vi "Write_Realim_Current.vi"(9 "Objetive Current":dbl, 11 "address string in":string) -> (1 "Boolean":bool, 3 "address string in 2":string)   [LabVIEW 2017]
panel:
  out "error out":errorcluster
  out "Numeric":i32
  out "Correction(x)":dbl
  out "Current":dbl[unit]
  out "Offset":dbl
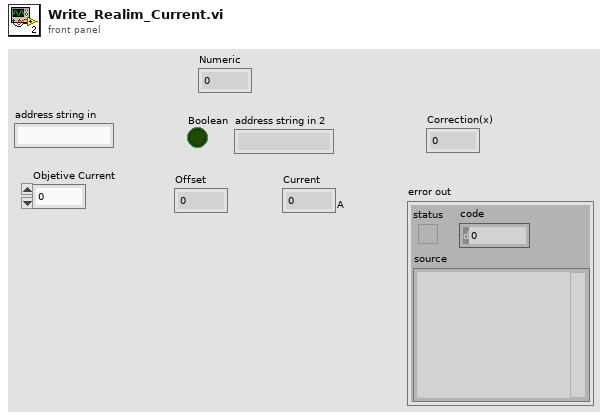
[diagram p1: front panel]
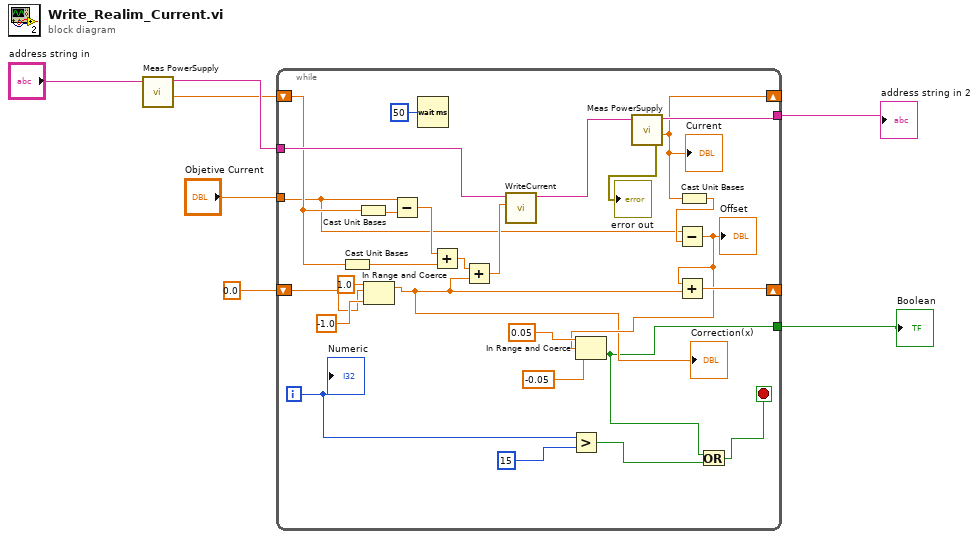
[diagram p0: block diagram]
diagram:
  n1 = call "Meas PowerSupply.vi"("address string"="address string in") -> ("address string 2"=w3:string, "Current"=w2:dbl[unit])  [unwired: 2 in, 2 out]
  n2 = while {
    tunnel: "Objetive Current" -> [w20]
    shift-right: [w23] -> _
    shift-left: 0.0 -> [w16]
    tunnel: [w11] -> w6
    tunnel: [w27] -> w5
    tunnel: w3 -> [w30]
    shift-right: [w26] -> _
    shift-left: w2 -> [w29]
    i -> [w10]
    stop <- w12 stop-if-true
    n3 = Cast Unit Bases(0:w29) -> (2:w33:dbl)  [unwired: 1 in]
    n4 = Cast Unit Bases(0:w29) -> (2:w34:dbl)  [unwired: 1 in]
    n5 = In Range and Coerce(upper limit=1.0, x=w16, lower limit=-1.0) -> (coerced(x)=w15:dbl)  [unwired: 1 out]
    "Correction(x)" <- w15
    n6 = Subtract(x=w20, y=w34) -> (x-y=w24:dbl)
    n7 = Wait (ms)(milliseconds to wait=u32 50) -> ()  [unwired: 1 out]
    n8 = Add(x=w24, y=w33) -> (x+y=w22:dbl)
    n9 = Add(x=w22, y=w15) -> (x+y=w21:dbl)
    n10 = call "WriteCurrent.vi"("Current"=w21, "address string in"=w30) -> ("address string in 2"=w28:string)  [unwired: 9 in]
    n11 = Greater?(x=w10, y=15) -> (0:w8:bool)
    n12 = call "Meas PowerSupply.vi"("address string"=w28) -> ("address string 2"=w27:string, "Current"=w26:dbl[unit], "error out"=→"error out":errorcluster)  [unwired: 2 in, 1 out]
    "Current" <- w26
    n13 = Cast Unit Bases(0:w26) -> (2:w25:dbl)  [unwired: 1 in]
    n14 = Subtract(x=w20, y=w25) -> (x-y=w19:dbl)
    "Offset" <- w19
    n15 = In Range and Coerce(upper limit=0.05, x=w19, lower limit=-0.05) -> (In Range?=w11:bool)  [unwired: 1 out]
    n16 = Add(x=w19, y=w15) -> (x+y=w23:dbl)
    n17 = Or(x=w11, y=w8) -> (x .or. y?=w12:bool)
    "Numeric" <- w10
  }
  "Boolean" <- w6
  "address string in 2" <- w5
